vi "Configure.vi"(6 "GridSize":u32, 7 "Mode":u32, 8 "error in (no error)":errorcluster, 9 "Save":bool, 11 "AODAcq in":refnum<class "AODAcq.lvclass">) -> (0 "error out":errorcluster, 3 "AODAcq out":refnum<class "AODAcq.lvclass">)   [LabVIEW 2014, in "AODAcq.lvclass"]
uses:
  AODAcq.lvclass
  AODAcq.lvclass/AODAcq.ctl
  <vilib>/Utility/error.llb/Error Cluster From Error Code.vi
  C:/Program Files (x86)/National Instruments/LabVIEW 2014/Targets/NI/FPGA/StockFPGA_IntfPrivate/ScriptTemplates/StockFPGA_PlugInRead32.vi
  <vilib>/rvi/errors/niLvFpgaAdjustHostInterfaceError.vi
  HDF5Tools/LabView/Create Dataset 2D Integer.vi
  HDF5Tools/LabView/Create Dataset 1D Double.vi
  HDF5Tools/LabView/Create Dataset 2D Double.vi
  <vilib>/rvi/interface/nirviReadWriteControl/nirviReadWriteControl.xnode
  FPGA_Control/AODRef.ctl
  FPGA Bitfiles/AodScanner_FPGATarget_AODControl(FPGA)_TyJc9yYmyGA.lvbitx
  HDF5Tools/LabView/HDF5Tools.lvlib
  NiFpgaLv.dll
  <vilib>/FPGAPlugInAG/PXIe-7965R/niLvFpga_Read32_PXIe-7965R.vi
  <vilib>/rvi/interface/nirviReadWriteControl/niFpgaRWControlAccessTimeoutTemplate.vi
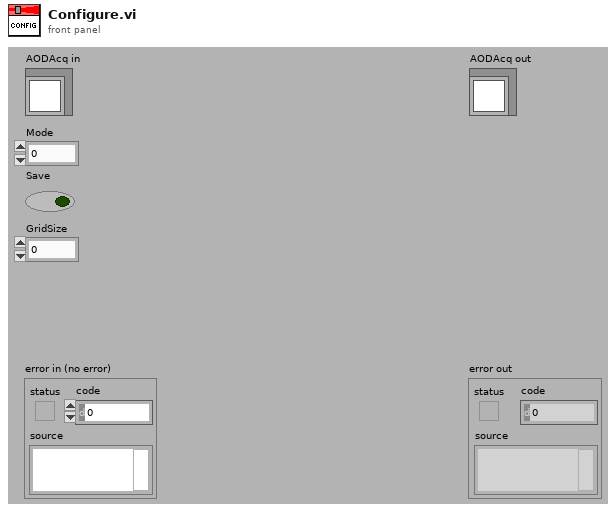
[diagram p1: front panel]
types:
  T1 = typedef "AODRef.ctl" = refnum<k20>
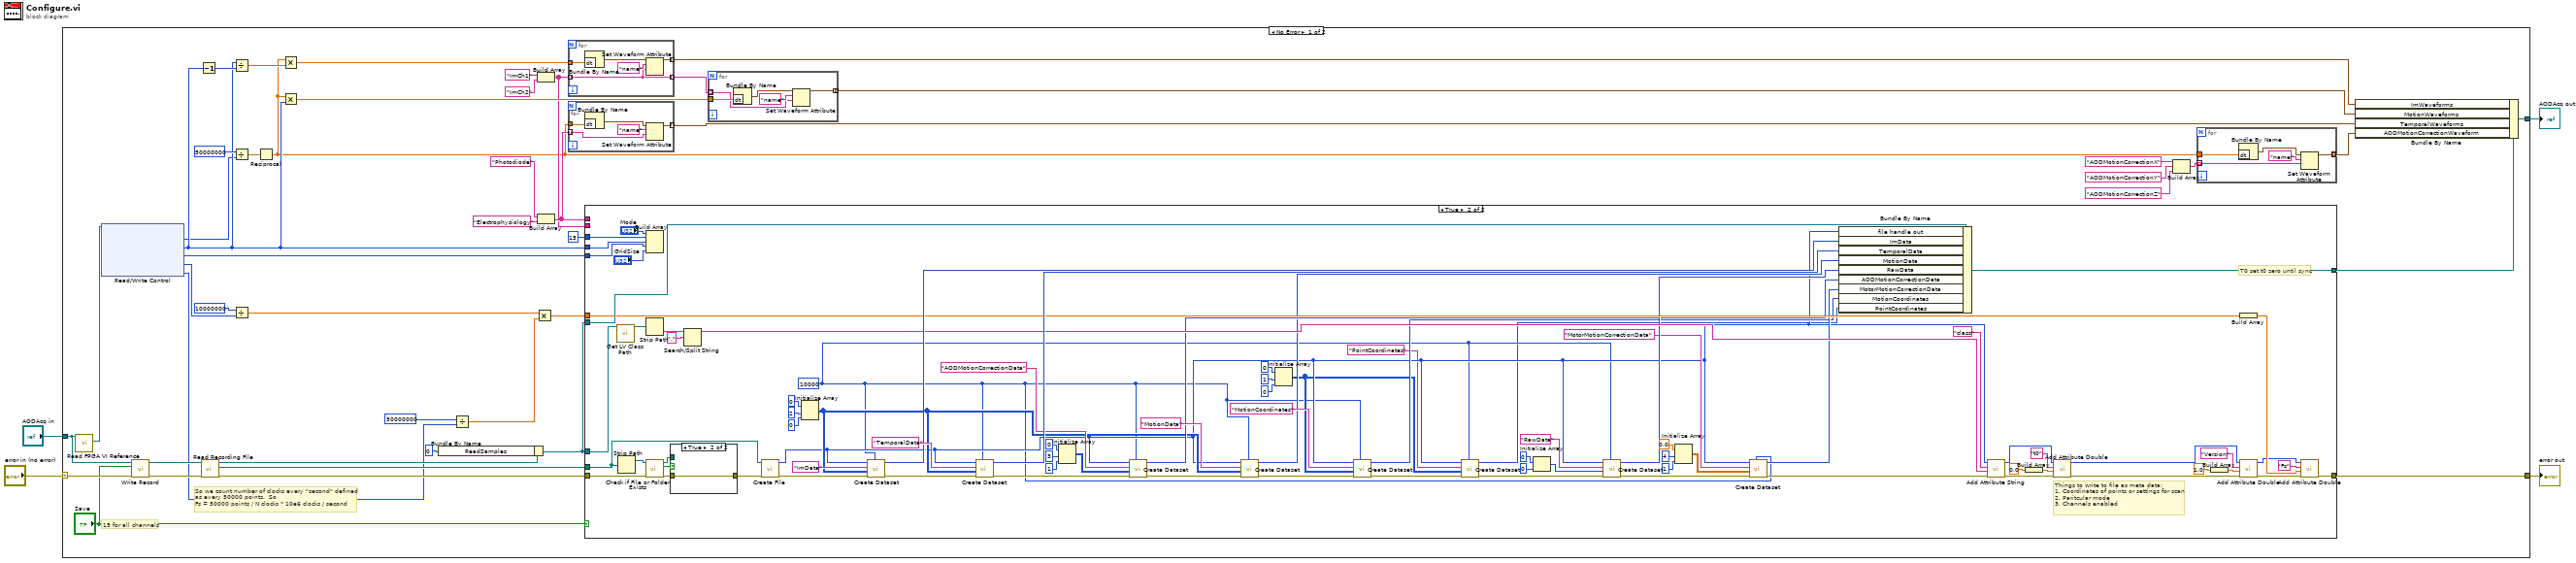
[diagram p0: block diagram]
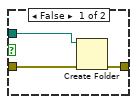
[diagram p3: hidden frame]
diagram:
  n1 = case shown="No Error" "error in (no error)" {
    selector: "error in (no error)" -> [w25 w161]
    tunnel: [w51 w161] -> w3
    tunnel: [w42 w160] -> w1
    tunnel: "AODAcq in" -> [w26 w160]
    frame No Error {
      # "So we count number of clocks every \"second\" defined\nas every 50000 points.  So\nFs = 50000 points / N clocks * 10e6 clocks / second"
      # "15 for all channels"
      n2 = call-dynamic "Read FPGA VI Reference.vi"("AODAcq in"=w26) -> ("FPGA VI Reference"=w45:T1)  [unwired: 8 in, 2 out]
      n3 = xnode "Read/Write Control"("FPGA VI Reference In"=w45) -> ("Setup.Downsample"=w27:u32, "Scan.Motion Increment"=w34:u32, "Scan.NumMotionPoints"=w33:u32, "Status.RelativeRate"=w17:u64, "Setup.Downsample"=w13:u32)  [unwired: 1 in, 2 out]
      n4 = call-dynamic "Write Record.vi"("error in (no error)"=w25, "Record"="Save", "AODAcq in"=w26) -> ("error out"=w22:errorcluster, "AODAcq out"=w23:refnum<class "AODAcq.lvclass">)  [unwired: 7 in]
      n5 = Decrement(x=w34) -> (x-1=w40:u32)
      n6 = call-dynamic "Read Recording File.vi"("error in (no error)"=w22, "AcquistionObject in"=w23) -> ("error out"=w19:errorcluster, "Recording File"=w21:path, "AcquistionObject out"=w20:refnum<class "AODAcq.lvclass">)  [unwired: 7 in]
      n7 = Divide(x=w34, y=w40) -> (x/y=w39:dbl)
      n8 = Divide(x=50000000, y=w27) -> (x/y=w47:dbl)
      n9 = Divide(x=u64 10000000 ("y"), y=w17) -> (x/y=w15:dbl)
      n10 = Reciprocal(x=w47) -> (1/x=w5:dbl)
      n11 = Multiply(x=w5, y=w39) -> (x*y=w41:dbl)
      n12 = Multiply(x=w5, y=w34) -> (x*y=w38:dbl)
      n13 = Bundle By Name(cluster=w20, "ReadSamples"=u64 0) -> (w18:refnum<class "AODAcq.lvclass">)
      n14 = Divide(x=u32 50000000, y=w13) -> (x/y=w11:dbl)
      n15 = Multiply(x=w15, y=w11) -> (x*y=w14:dbl)
      n16 = Build Array("ImCh1", "ImCh2") -> (w31:string[])
      n17 = Build Array("Photodiode", "Electrophysiology") -> (w32:string[])
      n18 = for {
        tunnel: w31 -> [w67] mode=indexing
        tunnel: w41 -> [w71]
        tunnel: [w68] -> w44 mode=indexing
        tunnel: [w67] -> w37 mode=indexing
        n19 = Bundle By Name("dt"=w71) -> (w70:waveform(dbl))  [unwired: 1 in]
        n20 = Set Waveform Attribute(5:w67, 6:"name" ("name"), 7:w70) -> (3:w68:waveform(dbl))  [unwired: 1 in, 2 out]
      }
      n21 = for {
        tunnel: w32 -> [w63] mode=indexing
        tunnel: w5 -> [w66]
        tunnel: [w62] -> w36 mode=indexing
        n22 = Bundle By Name("dt"=w66) -> (w65:waveform(dbl))  [unwired: 1 in]
        n23 = Set Waveform Attribute(5:w63, 6:"name" ("name"), 7:w65) -> (3:w62:waveform(dbl))  [unwired: 1 in, 2 out]
      }
      n24 = case shown="True" "Save" {
        tunnel: w21 -> [_ w138]
        tunnel: w18 -> [w73 w154]
        tunnel: [w73 w153] -> w43
        tunnel: w19 -> [w72 w135]
        tunnel: [w72 w112] -> w51
        tunnel: w31 -> [_ _]
        tunnel: w32 -> [_ _]
        tunnel: w34 -> [_ w151]
        tunnel: w33 -> [_ w152]
        tunnel: u32 15 -> [_ w150]
        tunnel: w18 -> [_ w126]
        tunnel: w14 -> [_ w110]
        frame False {
        }
        frame True {
          w75 = 10000 ("Chunk size")
          # "T0 set t0 zero until sync"
          # "Things to write to file as meta data:\n1. Coordinates of points or settings for scan\n2. Paritcular mode\n3. Channels enabled"
          n25 = call <vilib>:"Get LV Class Path.vi"("object"=w126) -> ("class path"=w131:path)  [unwired: 9 in, 1 out]
          n26 = Strip Path(path=w138) -> (stripped path=w136:path)  [unwired: 1 out]
          n27 = Build Array("Mode", w150, w151, w152, "GridSize") -> ()  [unwired: 1 out]
          n28 = Strip Path(path=w131) -> (name=w130:string)  [unwired: 1 out]
          n29 = call <vilib>:"Check if File or Folder Exists.vi"("error in (no error)"=w135, "path"=w136) -> ("error out"=w134:errorcluster, "file or folder exists?"=w133:bool, "dup path"=w132:path)  [unwired: 7 in]
          n30 = case shown="True" w133 {
            tunnel: [w158 w159] -> w137
            tunnel: w134 -> [w157 w159]
            tunnel: w132 -> [w156 _]
            frame False {
              n31 = Create Folder(path (use dialog)=w156, error in=w157) -> (error out=w158:errorcluster)  [unwired: 1 in, 2 out]
            }
            frame True {
            }
          }
          n32 = Search/Split String(string=w130, search string/char (-)=".") -> (substring before match=w128:string)  [unwired: 1 in, 2 out]
          n33 = call "Create File.vi"("Error in"=w137, "File Name"=w138) -> ("Error out"=w143:errorcluster, "file_id"=w80:i32)  [unwired: 6 in]
          n34 = Initialize Array(0, 2 ("dimension size"), 0 ("dimension size")) -> (w97:i32[][])
          n35 = call-poly "Create Dataset.vi"("Chunk size"=w75, "error in (no error)"=w143, "Datatype"=w97, "Dataset name"="ImData", "Location id in"=w80) -> ("error out"=w142:errorcluster, "Dataset id"=w141:i32)  [unwired: 5 in]
          n36 = call-poly "Create Dataset.vi"("Chunk size"=w75, "error in (no error)"=w142, "Datatype"=w97, "Dataset name"="TemporalData", "Location id in"=w80) -> ("error out"=w104:errorcluster, "Dataset id"=w140:i32)  [unwired: 5 in]
          n37 = Initialize Array(0 ("element"), 3 ("dimension size"), 1 ("dimension size")) -> (w91:i32[][])
          n38 = call-poly "Create Dataset.vi"("Chunk size"=w75, "error in (no error)"=w104, "Datatype"=w91, "Dataset name"="AODMotionCorrectionData", "Location id in"=w80) -> ("error out"=w103:errorcluster, "Dataset id"=w101:i32)  [unwired: 5 in]
          n39 = call-poly "Create Dataset.vi"("Chunk size"=w75, "error in (no error)"=w103, "Datatype"=w97, "Dataset name"="MotionData", "Location id in"=w80) -> ("error out"=w84:errorcluster, "Dataset id"=w83:i32)  [unwired: 5 in]
          n40 = Initialize Array(0 ("element"), 1 ("dimension size"), 0 ("dimension size")) -> (w78:i32[][])
          n41 = call-poly "Create Dataset.vi"("Chunk size"=w75, "error in (no error)"=w84, "Datatype"=w78, "Dataset name"="MotionCoordinates", "Location id in"=w80) -> ("error out"=w77:errorcluster, "Dataset id"=w82:i32)  [unwired: 5 in]
          n42 = call-poly "Create Dataset.vi"("Chunk size"=w75, "error in (no error)"=w77, "Datatype"=w78, "Dataset name"="PointCoordinates", "Location id in"=w80) -> ("error out"=w76:errorcluster, "Dataset id"=w74:i32)  [unwired: 5 in]
          n43 = Initialize Array(0, 0 ("dimension size")) -> (w106:i32[])
          n44 = call-poly "Create Dataset.vi"("Chunk size"=w75, "error in (no error)"=w76, "Datatype"=w106, "Dataset name"="RawData", "Location id in"=w80) -> ("error out"=w89:errorcluster, "dataset_id"=w105:i32)  [unwired: 5 in]
          n45 = Initialize Array(0.0 ("element"), 4 ("dimension size"), 1 ("dimension size")) -> (w95:dbl[][])
          n46 = call-poly "Create Dataset.vi"("Chunk size"=w75, "error in (no error)"=w89, "Datatype"=w95, "Dataset name"="MotorMotionCorrectionData", "Location id in"=w80) -> ("error out"=w98:errorcluster, "Dataset id"=w99:i32)  [unwired: 5 in]
          n47 = Bundle By Name(cluster=w154, "file handle out"=w80, "ImData"=w141, "TemporalData"=w140, "MotionData"=w83, "RawData"=w105, "AODMotionCorrectionData"=w101, "MotorMotionCorrectionData"=w99, "MotionCoordinates"=w82, "PointCoordinates"=w74) -> (w153:refnum<class "AODAcq.lvclass">)
          n48 = call "Add Attribute String.vi"("error in (no error)"=w98, "Attribute data"=w128, "Attribute name"="class", "loc_id"=w80) -> ("error out"=w122:errorcluster, "loc_id_out"=w121:i32)  [unwired: 6 in]
          n49 = Build Array(0.0 ("element")) -> (w124:dbl[])
          n50 = call "Add Attribute Double.vi"("error in (no error)"=w122, "data"=w124, "Attribute name"="t0", "loc_id"=w121) -> ("error out"=w117:errorcluster, "loc_id_out"=w116:i32)  [unwired: 6 in]
          n51 = Build Array(1.0) -> (w118:dbl[])
          n52 = Build Array(w110) -> (w115:dbl[])
          n53 = call "Add Attribute Double.vi"("error in (no error)"=w117, "data"=w118, "Attribute name"="Version", "loc_id"=w116) -> ("error out"=w114:errorcluster, "loc_id_out"=w113:i32)  [unwired: 6 in]
          n54 = call "Add Attribute Double.vi"("error in (no error)"=w114, "data"=w115, "Attribute name"="Fs", "loc_id"=w113) -> ("error out"=w112:errorcluster)  [unwired: 6 in, 1 out]
        }
      }
      n55 = for {
        tunnel: w37 -> [w58] mode=indexing
        tunnel: w38 -> [w61]
        tunnel: [w57] -> w35 mode=indexing
        n56 = Bundle By Name("dt"=w61) -> (w60:waveform(dbl))  [unwired: 1 in]
        n57 = Set Waveform Attribute(5:w58, 6:"name" ("name"), 7:w60) -> (3:w57:waveform(dbl))  [unwired: 1 in, 2 out]
      }
      n58 = Build Array("AODMotionCorrectionX", "AODMotionCorrectionY", "AODMotionCorrectionZ") -> (w7:string[])
      n59 = for {
        tunnel: w7 -> [w53] mode=indexing
        tunnel: w5 -> [w56]
        tunnel: [w52] -> w10 mode=indexing
        n60 = Bundle By Name("dt"=w56) -> (w55:waveform(dbl))  [unwired: 1 in]
        n61 = Set Waveform Attribute(5:w53, 6:"name" ("name"), 7:w55) -> (3:w52:waveform(dbl))  [unwired: 1 in, 2 out]
      }
      n62 = Bundle By Name(cluster=w43, "ImWaveforms"=w44, "MotionWaveforms"=w35, "TemporalWaveforms"=w36, "AODMotionCorrectionWaveform"=w10) -> (w42:refnum<class "AODAcq.lvclass">)
    }
    frame Error {
    }
  }
  "error out" <- w3
  "AODAcq out" <- w1
